vi "Target.vi"   [LabVIEW 2025]
uses:
  <vilib>/eio/utilities/niEioResolveVilibRelativePath.vi
  <vilib>/rvi/interface/RandomDataEmulation/niFpgaRandomDataHandleErrors.vi
  <vilib>/rvi/DataTransferAndStorage/Container/XNode/niFpgaContainer.xnode
  <vilib>/rvi/interface/RandomDataEmulation/nirviRandomDataFpgaReadWriteTemplate.vi
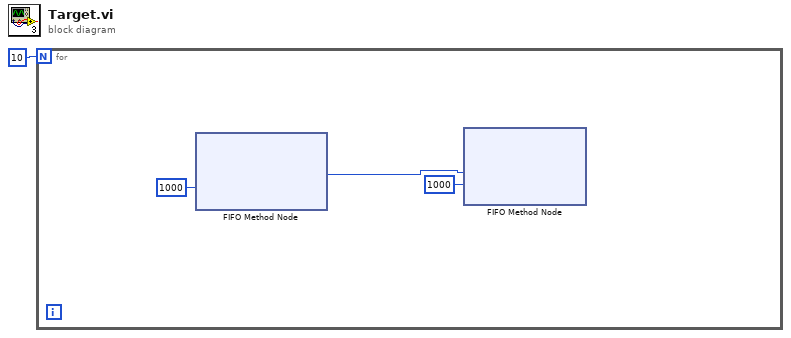
[diagram p0: block diagram]
diagram:
  n1 = for {
    N: 10 -> [_]
    n2 = xnode ("FIFO Method Node")("Timeout"=1000) -> ("Element"=w2:i32)  [unwired: 1 in, 2 out]
    n3 = xnode ("FIFO Method Node")("Element"=w2, "Timeout"=1000) -> ()  [unwired: 1 in, 2 out]
  }
